vi "Get_Sub_Collection.vi"(8 "error in (no error)":errorcluster caption="entrée d'erreur (pas d'erreur)", 11 "Firebase Benches en entrée":refnum<class "Firebase Scan.lvclass">) -> (0 "error out":errorcluster caption="sortie d'erreur", 3 "Firebase Benches en sortie":refnum<class "Firebase Scan.lvclass">)   [LabVIEW 2020, in "Library Instrument & Equipement.lvlib" / "Library FireBase.lvlib" / "Firebase Scan.lvclass"]
doc: "Return the documents present in the test collection for each DATA read with Get_Data\nPlease initialise the following values\n - Name BDD\n - Document of test sequence\n - API Key\n - Nb To Read"
uses:
  Firebase Scan.lvclass
  C:/Users/ngarcin/OneDrive - Altyor/Standard TB/Class/Firebase/Source/Firebase Driver/Firebase Driver.lvclass
  Firebase Scan.lvclass/Firebase Scan.ctl
  JSON API/JSON Value/Set from JSON string.vi
  JSON API/JSON Value/JSON Value.lvclass
  Firebase Altyor/Firebase Altyor.lvclass
  JSON API/Variant JSON/Variant JSON.lvlib
  JSON API/Get Polymorphic/JSON GetSet.lvlib
  Firebase Driver/Firebase Driver.lvclass
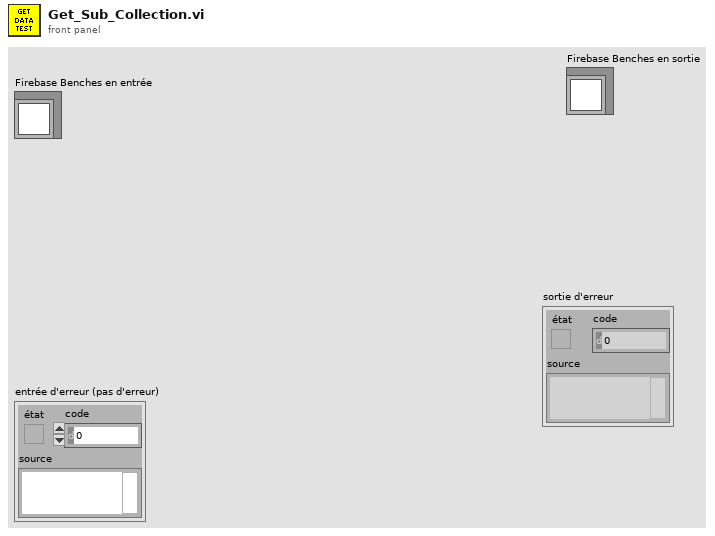
[diagram p1: front panel]
types:
  T1 = cluster{"documents":cluster{"name":string, "fields":cluster{"Result":cluster{"booleanValue":bool}, "CreationDate":cluster{"timestampValue":string}, "Batch":cluster{"stringValue":string}, "SerialNumber":cluster{"stringValue":string}, "EndOfProduction":cluster{"timestampValue":string}, "FW_Version":cluster{"mapValue":cluster{"fields":cluster{"Bootloader":cluster{"mapValue":cluster{"fields":cluster{"File_Name":cluster{"stringValue":string}, "Version":cluster{"mapValue":cluster{"fields":cluster{"Major":cluster{"stringValue":string}, "Minor":cluster{"stringValue":string}}}}, "Checksum":cluster{"stringValue":string}}}}, "SoftDevice":cluster{"mapValue":cluster{"fields":cluster{"File_Name":cluster{"stringValue":string}, "Version":cluster{"mapValue":cluster{"fields":cluster{"Major":cluster{"stringValue":string}, "Minor":cluster{"stringValue":string}}}}, "Checksum":cluster{"stringValue":string}}}}, "DFU":cluster{"mapValue":cluster{"fields":cluster{"File_Name":cluster{"stringValue":string}, "Version":cluster{"mapValue":cluster{"fields":cluster{"Major":cluster{"stringValue":string}, "Minor":cluster{"stringValue":string}}}}, "Checksum":cluster{"stringValue":string}}}}}}}, "PartNumber":cluster{"stringValue":string}, "OrderNumber":cluster{"stringValue":string}, "Operator":cluster{"stringValue":string}, "Deleted":cluster{"booleanValue":bool}}}[]}
  T2 = cluster{"name":string, "fields":cluster{"Result":cluster{"booleanValue":bool}, "Name":cluster{"stringValue":string}, "StartOfTest":cluster{"timestampValue":string}, "EndOfTest":cluster{"timestampValue":string}, "limit":cluster{"mapValue":cluster{"fields":cluster{"Lower":cluster{"stringValue":string}, "Upper":cluster{"stringValue":string}}}}, "Value":cluster{"stringValue":string}, "Type":cluster{"stringValue":string}, "MainTest":cluster{"stringValue":string}}}[][]
  T3 = cluster{"name":string, "fields":cluster{"Result":cluster{"booleanValue":bool}, "CreationDate":cluster{"timestampValue":string}, "Batch":cluster{"stringValue":string}, "SerialNumber":cluster{"stringValue":string}, "EndOfProduction":cluster{"timestampValue":string}, "FW_Version":cluster{"mapValue":cluster{"fields":cluster{"Bootloader":cluster{"mapValue":cluster{"fields":cluster{"File_Name":cluster{"stringValue":string}, "Version":cluster{"mapValue":cluster{"fields":cluster{"Major":cluster{"stringValue":string}, "Minor":cluster{"stringValue":string}}}}, "Checksum":cluster{"stringValue":string}}}}, "SoftDevice":cluster{"mapValue":cluster{"fields":cluster{"File_Name":cluster{"stringValue":string}, "Version":cluster{"mapValue":cluster{"fields":cluster{"Major":cluster{"stringValue":string}, "Minor":cluster{"stringValue":string}}}}, "Checksum":cluster{"stringValue":string}}}}, "DFU":cluster{"mapValue":cluster{"fields":cluster{"File_Name":cluster{"stringValue":string}, "Version":cluster{"mapValue":cluster{"fields":cluster{"Major":cluster{"stringValue":string}, "Minor":cluster{"stringValue":string}}}}, "Checksum":cluster{"stringValue":string}}}}}}}, "PartNumber":cluster{"stringValue":string}, "OrderNumber":cluster{"stringValue":string}, "Operator":cluster{"stringValue":string}, "Deleted":cluster{"booleanValue":bool}}}[]
  T4 = cluster{"name":string, "fields":cluster{"Result":cluster{"booleanValue":bool}, "Name":cluster{"stringValue":string}, "StartOfTest":cluster{"timestampValue":string}, "EndOfTest":cluster{"timestampValue":string}, "limit":cluster{"mapValue":cluster{"fields":cluster{"Lower":cluster{"stringValue":string}, "Upper":cluster{"stringValue":string}}}}, "Value":cluster{"stringValue":string}, "Type":cluster{"stringValue":string}, "MainTest":cluster{"stringValue":string}}}[]
  T5 = cluster{"documents":cluster{"name":string, "fields":cluster{"Result":cluster{"booleanValue":bool}, "Name":cluster{"stringValue":string}, "StartOfTest":cluster{"timestampValue":string}, "EndOfTest":cluster{"timestampValue":string}, "limit":cluster{"mapValue":cluster{"fields":cluster{"Lower":cluster{"stringValue":string}, "Upper":cluster{"stringValue":string}}}}, "Value":cluster{"stringValue":string}, "Type":cluster{"stringValue":string}, "MainTest":cluster{"stringValue":string}}}[], "nextPageToken":string}
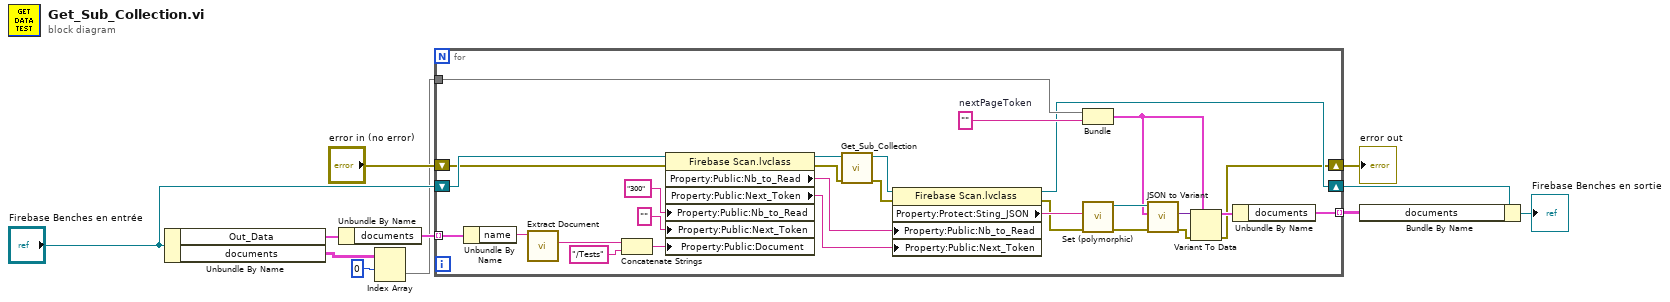
[diagram p0: block diagram]
diagram:
  n1 = Unbundle By Name("Firebase Benches en entrée") -> ("Out_Data"=w11:T1, "documents"=w4:T2)
  n2 = Unbundle By Name(w11) -> ("documents"=w10:T3)
  n3 = Index Array(array=w4, index (row)=0 ("indice (ligne)")) -> (element=w3:T4)  [unwired: 1 in]
  n4 = for {
    tunnel: [w32] -> w6 mode=indexing
    shift-right: [w13] -> w1
    shift-left: "Firebase Benches en entrée" -> [w31]
    shift-right: [w12] -> w9
    shift-left: "error in (no error)" -> [w30]
    tunnel: w10 -> [w29] mode=indexing
    tunnel: w3 -> [w16]
    w34 = ""  # nextPageToken
    n5 = Unbundle By Name(w29) -> ("name"=w28:string)
    n6 = call "Extract Document.vi"("Name"=w28) -> ("Source"=w27:string)  [unwired: 9 in, 1 out]
    n7 = Concatenate Strings(w27, "/Tests" ("chaîne")) -> (w25:string)
    n8 = property class="Firebase Scan.lvclass"(reference=w31, error in=w30, "Property:Public:Nb_to_Read"="300" ("Nb_to_Read"), "Property:Public:Next_Token"="" ("Next_Token"), "Property:Public:Document"=w25) -> (reference out=w17:refnum<class "Firebase Scan.lvclass">, error out=w20:errorcluster, "Property:Public:Nb_to_Read"=w24:string, "Property:Public:Next_Token"=w22:string)
    n9 = call-parent "Get_Sub_Collection.vi"("error in (no error)"=w20, "Firebase Altyor en entrée"=w17) -> ("error out"=w19:errorcluster, "Firebase Altyor en sortie"=w18:refnum<class "Firebase Scan.lvclass">)  [unwired: 8 in]
    n10 = property class="Firebase Scan.lvclass"(reference=w18, error in=w19, "Property:Public:Nb_to_Read"=w24, "Property:Public:Next_Token"=w22) -> (reference out=w13:refnum<class "Firebase Scan.lvclass">, error out=w15:errorcluster, "Property:Protect:Sting_JSON"=w36:string)
    n11 = Bundle("documents"=w16, "nextPageToken"=w34) -> (w33:T5)  [unwired: 1 in]
    n12 = call-poly "Set (polymorphic).vi"("error in (no error)"=w15, "JSON stream"=w36) -> ("error out"=w37:errorcluster, "JSON Value out"=w39:refnum<class "JSON Value.lvclass">)  [unwired: 7 in, 1 out]
    n13 = call "JSON to Variant.vi"("error in (no error)"=w37, "Variant (Data Type)"=w33, "JSON Value"=w39) -> ("error out"=w38:errorcluster, "Variant out"=w14:variant)  [unwired: 7 in]
    n14 = Variant To Data(error in=w38, type=w33, Variant=w14) -> (data=w35:T5, error out=w12:errorcluster)
    n15 = Unbundle By Name(w35) -> ("documents"=w32:T4)
  }
  "error out" <- w9
  n16 = Bundle By Name(cluster=w1, "documents"=w6) -> (→"Firebase Benches en sortie":refnum<class "Firebase Scan.lvclass">)
